vi "CMD_11T_Enable_Heater.vi"(11 "VISA resource name":refnum<visa-resource-name>) -> (3 "VISA resource name out":refnum<visa-resource-name>)   [LabVIEW 2013]
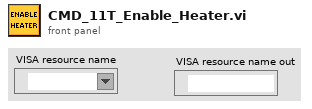
[diagram p1: front panel]
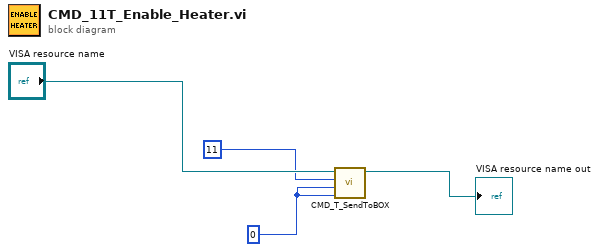
[diagram p0: block diagram]
diagram:
  w2 = i16 0 ("arg2")
  n1 = call "CMD_T_SendToBOX.vi"("arg2"=w2, "arg1"=w2, "CMD"=i8 11, "VISA resource name"="VISA resource name") -> ("VISA resource name out"=→"VISA resource name out":refnum<visa-resource-name>)  [unwired: 7 in]
